vi "SR_J-Read Joystick.vi"(8 "error in (no error)":errorcluster, 10 "RDS Msg Q in":refnum<user-event>, 11 "Joystick":T1) -> (0 "error out":errorcluster, 2 "RDS Msg Q out":refnum<user-event>, 3 "Joystick Out":T1)   [LabVIEW 2015, in "Shore Library.lvlib"]
uses:
  Shore Library.lvlib
  SR-J-State.ctl
  Libraries/RDS Framework/RDS Message Class/RDS Message.lvclass
  <vilib>/Utility/inputDevices.llb/joystickAcquire.vi
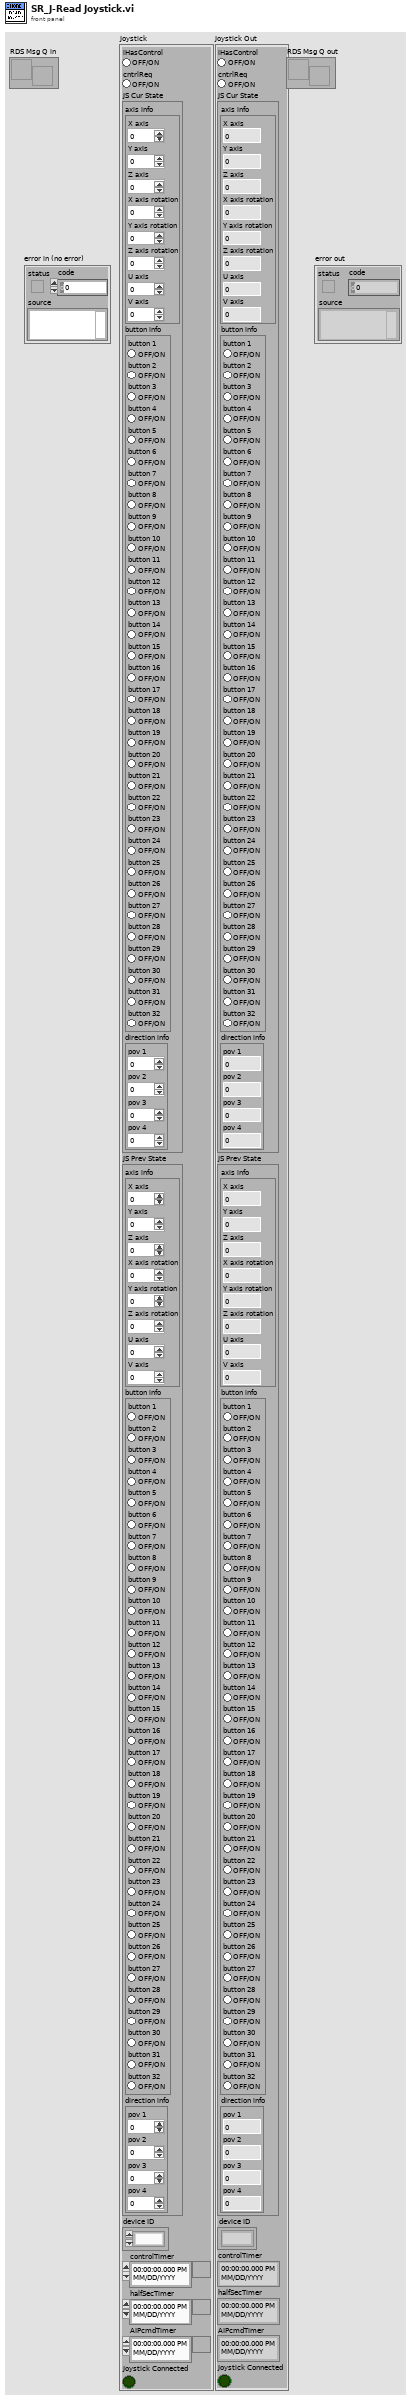
[diagram p1: front panel]
types:
  T1 = typedef "Shore Library.lvlib/SR-J-State.ctl" = cluster{"iHasControl":bool, "cntrlReq":bool, "JS Cur State":cluster{"axis info":cluster{"X axis":i32, "Y axis":i32, "Z axis":i32, "X axis rotation":i32, "Y axis rotation":i32, "Z axis rotation":i32, "U axis":i32, "V axis":i32}, "button info":cluster{"button 1":bool, "button 2":bool, "button 3":bool, "button 4":bool, "button 5":bool, "button 6":bool, "button 7":bool, "button 8":bool, "button 9":bool, "button 10":bool, "button 11":bool, "button 12":bool, "button 13":bool, "button 14":bool, "button 15":bool, "button 16":bool, "button 17":bool, "button 18":bool, "button 19":bool, "button 20":bool, "button 21":bool, "button 22":bool, "button 23":bool, "button 24":bool, "button 25":bool, "button 26":bool, "button 27":bool, "button 28":bool, "button 29":bool, "button 30":bool, "button 31":bool, "button 32":bool}, "direction info":cluster{"pov 1":i32, "pov 2":i32, "pov 3":i32, "pov 4":i32}}, "JS Prev State":cluster{"axis info":cluster{"X axis":i32, "Y axis":i32, "Z axis":i32, "X axis rotation":i32, "Y axis rotation":i32, "Z axis rotation":i32, "U axis":i32, "V axis":i32}, "button info":cluster{"button 1":bool, "button 2":bool, "button 3":bool, "button 4":bool, "button 5":bool, "button 6":bool, "button 7":bool, "button 8":bool, "button 9":bool, "button 10":bool, "button 11":bool, "button 12":bool, "button 13":bool, "button 14":bool, "button 15":bool, "button 16":bool, "button 17":bool, "button 18":bool, "button 19":bool, "button 20":bool, "button 21":bool, "button 22":bool, "button 23":bool, "button 24":bool, "button 25":bool, "button 26":bool, "button 27":bool, "button 28":bool, "button 29":bool, "button 30":bool, "button 31":bool, "button 32":bool}, "direction info":cluster{"pov 1":i32, "pov 2":i32, "pov 3":i32, "pov 4":i32}}, "device ID":refnum<k1>, "controlTimer":timestamp, "halfSecTimer":timestamp, "AIPcmdTimer":timestamp, "Joystick Connected":bool}
  T2 = cluster{"X axis":i32, "Y axis":i32, "Z axis":i32, "X axis rotation":i32, "Y axis rotation":i32, "Z axis rotation":i32, "U axis":i32, "V axis":i32}
  T3 = cluster{"button 1":bool, "button 2":bool, "button 3":bool, "button 4":bool, "button 5":bool, "button 6":bool, "button 7":bool, "button 8":bool, "button 9":bool, "button 10":bool, "button 11":bool, "button 12":bool, "button 13":bool, "button 14":bool, "button 15":bool, "button 16":bool, "button 17":bool, "button 18":bool, "button 19":bool, "button 20":bool, "button 21":bool, "button 22":bool, "button 23":bool, "button 24":bool, "button 25":bool, "button 26":bool, "button 27":bool, "button 28":bool, "button 29":bool, "button 30":bool, "button 31":bool, "button 32":bool}
  T4 = cluster{"pov 1":i32, "pov 2":i32, "pov 3":i32, "pov 4":i32}
  T5 = cluster{"axis info":cluster{"X axis":i32, "Y axis":i32, "Z axis":i32, "X axis rotation":i32, "Y axis rotation":i32, "Z axis rotation":i32, "U axis":i32, "V axis":i32}, "button info":cluster{"button 1":bool, "button 2":bool, "button 3":bool, "button 4":bool, "button 5":bool, "button 6":bool, "button 7":bool, "button 8":bool, "button 9":bool, "button 10":bool, "button 11":bool, "button 12":bool, "button 13":bool, "button 14":bool, "button 15":bool, "button 16":bool, "button 17":bool, "button 18":bool, "button 19":bool, "button 20":bool, "button 21":bool, "button 22":bool, "button 23":bool, "button 24":bool, "button 25":bool, "button 26":bool, "button 27":bool, "button 28":bool, "button 29":bool, "button 30":bool, "button 31":bool, "button 32":bool}, "direction info":cluster{"pov 1":i32, "pov 2":i32, "pov 3":i32, "pov 4":i32}}
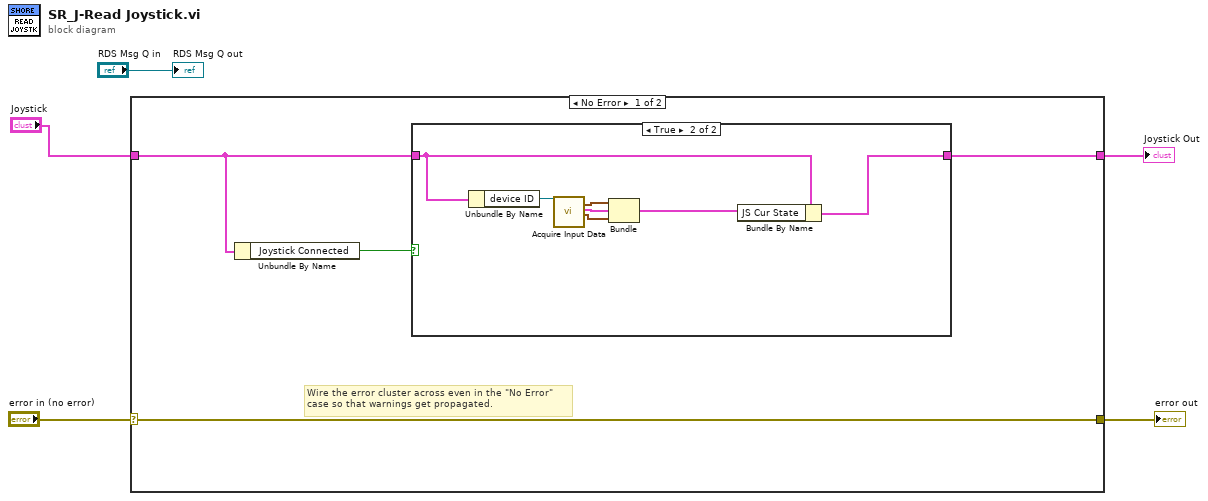
[diagram p0: block diagram]
diagram:
  n1 = case shown="No Error" "error in (no error)" {
    selector: "error in (no error)" -> [w9 w19]
    tunnel: [w9 w19] -> w4
    tunnel: [w8 w18] -> w2
    tunnel: "Joystick" -> [w7 w18]
    frame No Error {
      # "Wire the error cluster across even in the \"No Error\"\ncase so that warnings get propagated."
      n2 = Unbundle By Name(w7) -> ("Joystick Connected"=w6:bool)
      n3 = case shown="True" w6 {
        tunnel: w7 -> [w10 w13]
        tunnel: [w10 w12] -> w8
        frame False {
        }
        frame True {
          n4 = Unbundle By Name(w13) -> ("device ID"=w14:refnum<k1>)
          n5 = call-poly <vilib>:"Acquire Input Data.vi"("device ID"=w14) -> ("axis info"=w17:T2, "button info"=w16:T3, "direction info"=w15:T4)  [unwired: 1 in, 15 out]
          n6 = Bundle("axis info"=w17, "button info"=w16, "direction info"=w15) -> (w11:T5)  [unwired: 1 in]
          n7 = Bundle By Name(cluster=w13, "JS Cur State"=w11) -> (w12:T1)
        }
      }
    }
    frame Error {
    }
  }
  "error out" <- w4
  "Joystick Out" <- w2
  "RDS Msg Q out" <- "RDS Msg Q in"
